vi "Example Simple.vi"() -> ()   [LabVIEW 2010]
uses:
  C:/tf/play/labview/Tinkerforge.dll
  Tinkerforge.dll
panel:
  out "altitude (m)":sgl
  out "air pressure (mbar)":sgl
  in  "uid":string="jmQ"
  in  "port":i32=4223
  in  "host":string="localhost"
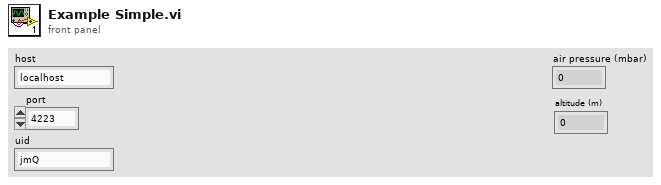
[diagram p1: front panel]
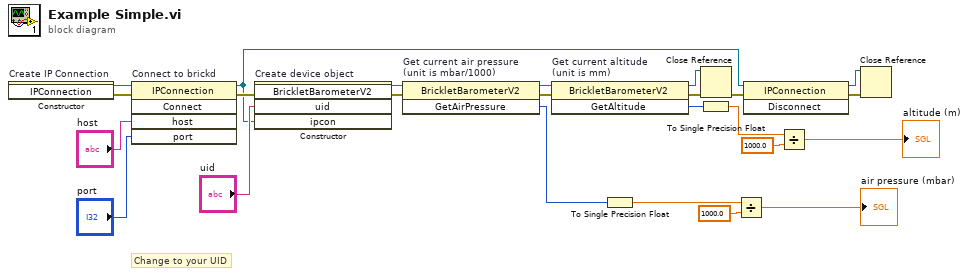
[diagram p0: block diagram]
diagram:
  # "Change to your UID"
  n1 = constructor on="Create IP Connection" class="IPConnection"() -> (reference out=w24:refnum<k24>, error out=w1:errorcluster)  [unwired: 3 in, 1 out]
  n2 = invoke on="Connect to brickd" class="IPConnection" method="Connect"(reference=w24, error in=w1, "host"="host", "port"="port") -> (reference out=w15:refnum<k24>, error out=w20:errorcluster)  [unwired: 1 in, 3 out]
  n3 = constructor on="Create device object" class="BrickletBarometerV2"(error in=w20, "uid"="uid", "ipcon"=w15) -> (reference out=w18:refnum<k24>, error out=w19:errorcluster)  [unwired: 2 in, 3 out]
  n4 = invoke on="Get current air pressure\n(unit is mbar/1000)" class="BrickletBarometerV2" method="GetAirPressure"(reference=w18, error in=w19) -> (reference out=w4:refnum<k24>, error out=w5:errorcluster, "GetAirPressure"=w13:i32)  [unwired: 1 in]
  n5 = invoke on="Get current altitude\n(unit is mm)" class="BrickletBarometerV2" method="GetAltitude"(reference=w4, error in=w5) -> (reference out=w2:refnum<k24>, error out=w3:errorcluster, "GetAltitude"=w9:i32)  [unwired: 1 in]
  n6 = To Single Precision Float(number=w13) -> (single precision float=w11:sgl)
  n7 = Close Reference(reference=w2, error in (no error)=w3) -> (error out=w17:errorcluster)
  n8 = To Single Precision Float(number=w9) -> (single precision float=w7:sgl)
  n9 = Divide(x=w11, y=sgl 1000.0) -> (x/y=→"air pressure (mbar)":sgl)
  n10 = invoke class="IPConnection" method="Disconnect"(reference=w15, error in=w17) -> (reference out=w14:refnum<k24>, error out=w16:errorcluster)  [unwired: 1 in, 1 out]
  n11 = Divide(x=w7, y=sgl 1000.0) -> (x/y=→"altitude (m)":sgl)
  n12 = Close Reference(reference=w14, error in (no error)=w16) -> ()  [unwired: 1 out]
